vi "题目7.vi"() -> ()   [LabVIEW 2017]
uses:
  <vilib>/Utility/miscctls.llb/LVBoundsTypeDef.ctl
  <vilib>/Utility/miscctls.llb/LVPositionTypeDef.ctl
panel:
  in  "键选中":bool
  in  "闪烁":bool
  in  "禁用":T1(ring)
  in  "停止":bool
  out "位置":T2
  out "边界":T3
  in  "可见":bool
  in  "数值":dbl
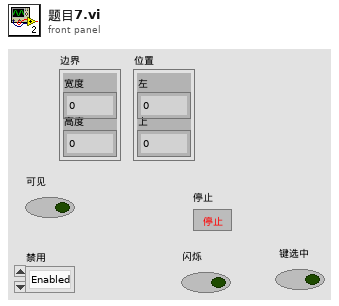
[diagram p1: front panel]
types:
  T1 = enum8{"Enabled", "Disabled", "Disabled and Grayed Out"}
  T2 = typedef "LVPositionTypeDef.ctl" = cluster{"Left":i32, "Top":i32}
  T3 = typedef "LVBoundsTypeDef.ctl" = cluster{"Width":u32, "Height":u32}
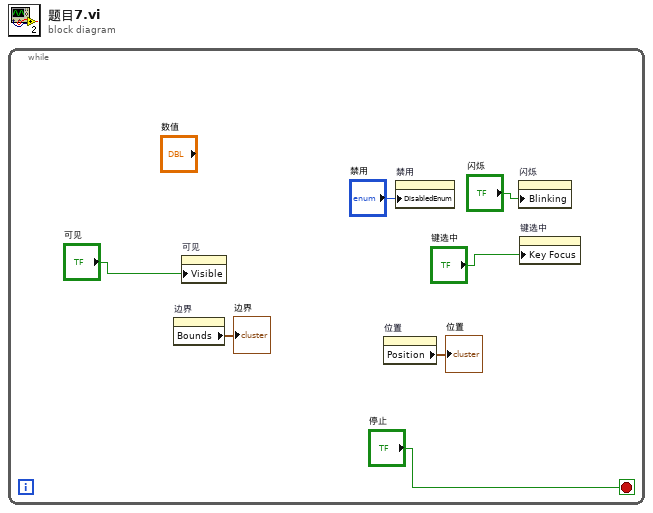
[diagram p0: block diagram]
diagram:
  n1 = while {
    stop <- "停止" stop-if-true
    n2 = property on="边界" class="DigNum (严格)"() -> ("Bounds"=→"边界":T3)  [unwired: 2 in, 2 out]
    n3 = property on="可见" class="DigNum (严格)"("Visible"="可见") -> ()  [unwired: 2 in, 2 out]
    n4 = property on="位置" class="DigNum (严格)"() -> ("Position"=→"位置":T2)  [unwired: 2 in, 2 out]
    n5 = property on="禁用" class="DigNum (严格)"("DisabledEnum"="禁用") -> ()  [unwired: 2 in, 2 out]
    n6 = property on="闪烁" class="DigNum (严格)"("Blinking"="闪烁") -> ()  [unwired: 2 in, 2 out]
    n7 = property on="键选中" class="DigNum (严格)"("Key Focus"="键选中") -> ()  [unwired: 2 in, 2 out]
  }
